vi "TestStand, Set Step from Table.vi"(8 "error in":errorcluster, 10 "Sequence Context":refnum<k7>, 11 "Tbl Refnum":refnum<vi>) -> (0 "error out":errorcluster, 2 "Sequence Context Out":refnum<k7>, 3 "Tbl Refnum out":refnum<vi>)   [LabVIEW 2010]
doc: "Transfers the information in a Test Criteria table to the current TestStand Sequence step for pass/fail evaluation by TestStand."
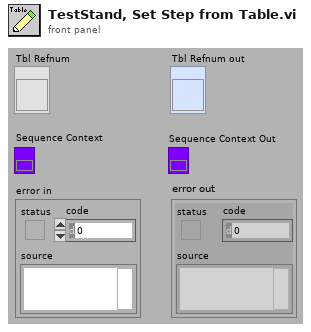
[diagram p1: front panel]
types:
  T1 = typedef "TestStand_Result Control.ctl" = cluster{"Measurement Name":string, "Result":dbl, "Low Limit":dbl, "High Limit":dbl, "Units":string, "Comp":string, "DataFmt":string, "LimitFmt":string}
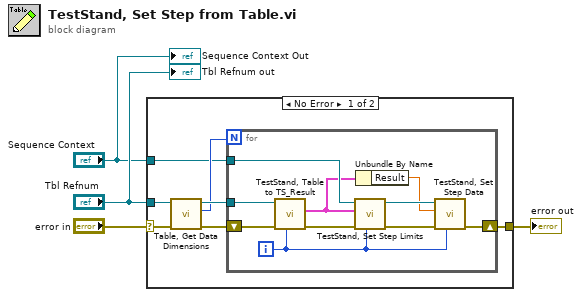
[diagram p0: block diagram]
diagram:
  n1 = case shown="No Error" "error in" {
    selector: "error in" -> [w5 w22]
    tunnel: [w11 w22] -> w4
    tunnel: "Sequence Context" -> [w6 _]
    tunnel: "Tbl Refnum" -> [w9 _]
    frame No Error {
      n2 = call "Table, Get Data Dimensions.vi"("error in"=w5, "Tbl Refnum"=w9) -> ("error out"=w10:errorcluster, "row_n"=w7:i32, "Tbl Refnum out"=w8:refnum<vi>)  [unwired: 6 in, 1 out]
      n3 = for {
        N: w7 -> [_]
        tunnel: w6 -> [w21]
        shift-right: [w19] -> w11
        shift-left: w10 -> [w16]
        tunnel: w8 -> [w12]
        i -> [w13]
        n4 = call "TestStand, Table to TS_Result.vi"("row (0)"=w13, "error in"=w16, "Tbl Refnum"=w12) -> ("error out"=w15:errorcluster, "TestStand Result"=w14:T1)  [unwired: 6 in, 1 out]
        n5 = call "TestStand, Set Step Limits.vi"("TS index"=w13, "error in"=w15, "CDT_type"=w14, "Sequence Context"=w21) -> ("error out"=w20:errorcluster, "Sequence Context Out"=w18:refnum<k7>)  [unwired: 6 in]
        n6 = Unbundle By Name(w14) -> ("Result"=w17:dbl)
        n7 = call "TestStand, Set Step Data.vi"("TS index"=w13, "error in"=w20, "Result"=w17, "Sequence Context"=w18) -> ("error out"=w19:errorcluster)  [unwired: 6 in, 1 out]
      }
    }
    frame Error {
    }
  }
  "error out" <- w4
  "Tbl Refnum out" <- "Tbl Refnum"
  "Sequence Context Out" <- "Sequence Context"
